vi "VectorCased3d.vi"(11 "XYUVArray":dbl[][](array[numeric])=[[-138.0, 28.0, -5.0, -3.0], [-92.0, 28.0, -10.0, -5.5], [-46.0, 28.0, -5.0, -10.5], [0.0, 28.0, -9.0, 3.5], [46.0, 28.0, -22.0, 1.0], [92.0, 28.0, -24.5, -9.0], [138.0, 28.0, -16.0, -23.0], [-138.0, 60.0, -6.0, -2.0], [-92.0, 60.0, -7.0, -12.0], [-46.0, 60.0, -6.0, -11.0], [0.0, 60.0, -9.0, 3.0], [46.0, 60.0, -5.5, 6.0], [92.0, 60.0, -10.0, -7.5], [138.0, 60.0, -17.0, -22.0], [-138.0, 92.0, 0.5, 2.0], [-92.0, 92.0, -1.5, -15.0], [-46.0, 92.0, -1.5, -10.5], [0.0, 92.0, 1.0, -1.5], [46.0, 92.0, 1.0, 3.0], [92.0, 92.0, -2.5, -7.5], [138.0, 92.0, -5.0, -17.0], [-138.0, 124.0, 18.5, 15.0], [-92.0, 124.0, 10.5, -2.5], [-46.0, 124.0, 6.5, -2.0], [0.0, 124.0, 7.5, 5.0], [46.0, 124.0, 9.5, 12.5], [92.0, 124.0, 14.0, 8.5], [138.0, 124.0, 6.5, -4.0], [-138.0, 156.0, 13.5, 14.5], [-92.0, 156.0, 19.5, 4.0], [-46.0, 156.0, 12.5, -1.0], [0.0, 156.0, 10.5, 3.5], [46.0, 156.0, 14.0, 11.0], [92.0, 156.0, 17.5, 10.5], [138.0, 156.0, 12.0, -4.5], [-138.0, 188.0, 9.0, 16.5], [-92.0, 188.0, 10.0, 8.0], [-46.0, 188.0, 14.0, 4.0], [0.0, 188.0, 15.5, 8.0], [46.0, 188.0, 14.5, 11.0], [92.0, 188.0, 21.5, 11.0], [138.0, 188.0, 19.0, 0.5], [-138.0, 214.0, 12.5, 11.5], [-92.0, 214.0, 17.5, 6.0], [-46.0, 214.0, 17.0, 9.5], [0.0, 214.0, 14.5, 10.5], [46.0, 214.0, 19.0, 10.5], [92.0, 214.0, 20.0, 7.0], [138.0, 214.0, 16.5, 7.0]]) -> ()   [LabVIEW 2020]
uses:
  <vilib>/Math Plots/3D Math Plots/3D Quiver/3D Quiver XCtrl/3D Quiver.xctl
  <vilib>/Math Plots/3D Math Plots/3D Quiver/3D Quiver Datatype/Public/Plot Helper (Matrix).vi
  <vilib>/Math Plots/3D Math Plots/3D Quiver/3D Quiver Datatype/3D Quiver Datatype.lvclass
panel:
  out "3D Quiver":refnum<class "3D Plot Datatype.lvclass">[](xcontrol)
  in  "stop":bool
  in  "VectorScale":dbl(slide)=1.5 min=0.0 step=0.25 scale=0.0..5.0
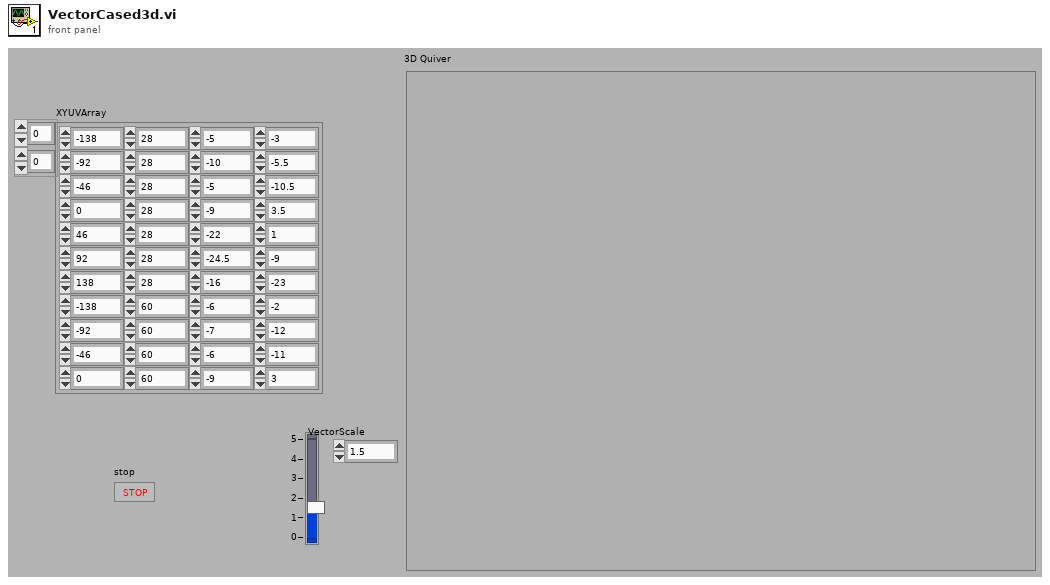
[diagram p1: front panel]
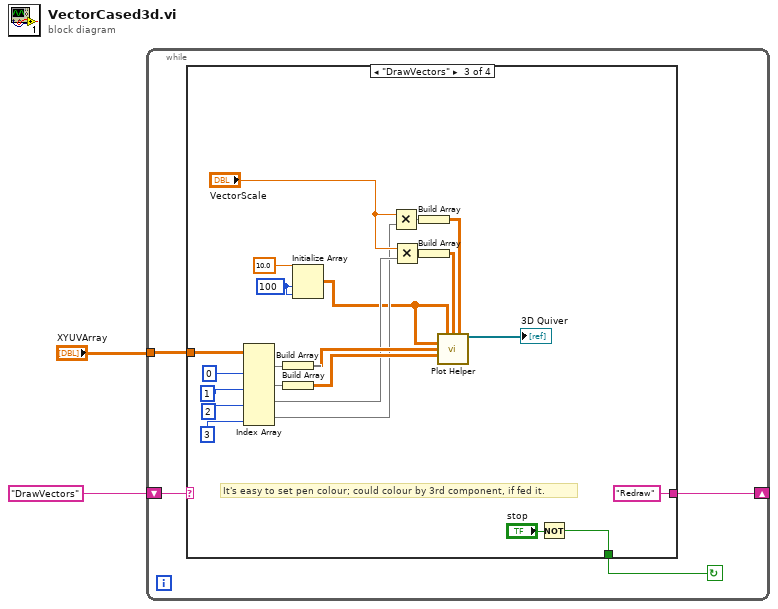
[diagram p0: block diagram]
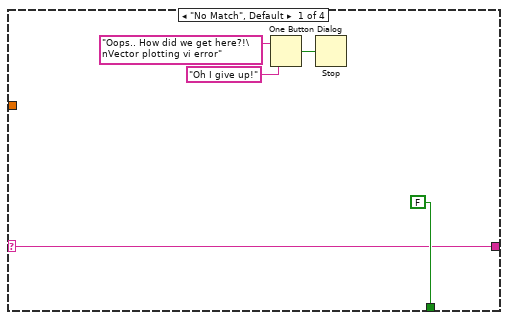
[diagram p2: hidden frame]
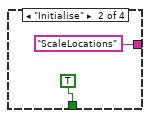
[diagram p3: hidden frame]
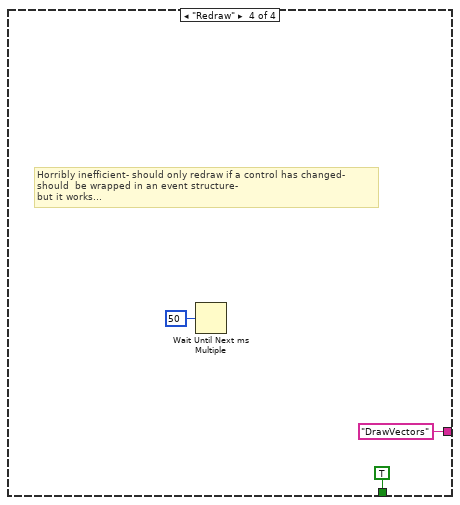
[diagram p4: hidden frame]
diagram:
  n1 = while {
    shift-right: [w3] -> _
    shift-left: "DrawVectors" -> [w6]
    tunnel: "XYUVArray" -> [w4]
    stop <- w5 continue-if-true
    n2 = case shown="\"DrawVectors\"" w6 {
      selector: w6 -> [w10 _ _ _]
      tunnel: [FALSE TRUE w34 TRUE] -> w5
      tunnel: w4 -> [_ _ w32 _]
      tunnel: [w10 "ScaleLocations" "Redraw" "DrawVectors"] -> w3
      frame "No Match", Default {
        n3 = One Button Dialog(message="Oops.. How did we get here?!\nVector plotting vi error", button name ("OK")="Oh I give up!") -> (true=w7:bool)
        n4 = Stop(stop? (T)=w7) -> ()
      }
      frame "Initialise" {
      }
      frame "DrawVectors" {
        w15 = 100 ("dimension size")
        # "It's easy to set pen colour; could colour by 3rd component, if fed it."
        n5 = Index Array(array=w32, index (col) #1=0 ("disabled index (col)"), index (col) #2=1 ("disabled index (col)"), index (col) #3=2 ("disabled index (col)"), index (col) #4=3 ("disabled index (col)")) -> (element #1=w31:dbl[], element #2=w29:dbl[], element #3=w23:dbl[], element #4=w19:dbl[])  [unwired: 4 in]
        n6 = Build Array(w31) -> (w30:dbl[][])
        n7 = Build Array(w29) -> (w28:dbl[][])
        n8 = Initialize Array(10.0 ("element"), w15, w15) -> (w16:dbl[][])
        n9 = Multiply(x="VectorScale", y=w19) -> (x*y=w18:dbl[])
        n10 = Multiply(x="VectorScale", y=w23) -> (x*y=w22:dbl[])
        n11 = Build Array(w18) -> (w17:dbl[][])
        n12 = Build Array(w22) -> (w21:dbl[][])
        n13 = call-poly <vilib>:"Plot Helper.vi"("Nx matrix"=w16, "Ny matrix"=w21, "Nz matrix"=w17, "x matrix"=w16, "y matrix"=w30, "z matrix"=w28) -> ("3D Plot lvclass Array out"=→"3D Quiver":refnum<class "3D Plot Datatype.lvclass">[])  [unwired: 3 in, 6 out]
        n14 = Not(x="stop") -> (.not. x?=w34:bool)
      }
      frame "Redraw" {
        # "Horribly inefficient- should only redraw if a control has changed-\nshould  be wrapped in an event structure-\nbut it works..."
        n15 = Wait Until Next ms Multiple(millisecond multiple=u32 50) -> ()  [unwired: 1 out]
      }
    }
  }
